vi "Simulated VeriStand Engine.PCL.vi"(8 "error in (no error)":errorcluster, 11 "Simulated VeriStand Engine in":refnum<class "Simulated VeriStand Engine.lvclass">) -> (0 "error out":errorcluster, 3 "Simulated VeriStand Engine out":refnum<class "Simulated VeriStand Engine.lvclass">)   [LabVIEW 2016, in "Simulated VeriStand Engine.lvclass"]
uses:
  Simulated VeriStand Engine.lvclass
  Simulated VeriStand Engine.lvclass/Simulated VeriStand Engine.ctl
  Simulated VeriStand Engine Interface/Simulated VeriStand Engine.Interface.lvclass/Simulated VeriStand Engine.Interface.ctl
  Source/Submodules/Memory/Source/Classes/Pointer/Memory.Pointer.lvclass/Memory.Pointer.ctl
  Accessors/Simulated VeriStand Engine.Get Interface.vi
  Simulated VeriStand Engine Interface/Methods/Simulated VeriStand Engine.Interface.Read.vi
  Simulated VeriStand Engine Interface/Methods/Simulated VeriStand Engine.Interface.Read.Stop.vi
  Source/Submodules/Memory/Source/Classes/Pointer/Memory.Pointer.Read.vi
  Source/Submodules/Memory/Source/Classes/Pointer/Memory.Pointer.Read.Safe.0D.Bool.vi
  Simulated VeriStand Engine Interface/Accessors/Simulated VeriStand Engine.Interface.Get Pointers.vi
  Simulated VeriStand Engine Interface/Accessors/Simulated VeriStand Engine.Interface.Get Control Pointers.vi
  Source/Submodules/Memory/Source/Classes/Pointer/Memory.Pointer.Read.Unsafe.0D.Bool.vi
  Source/Submodules/Memory/Source/Classes/Pointer/Memory.Pointer.Parameter Check.Null Pointer.vi
  Source/Submodules/Memory/Source/Classes/Pointer/Memory.Pointer.Parameter Check.Subset.vi
  Source/Submodules/Memory/Source/Classes/Pointer/Memory.Pointer.Get Address.vi
  Source/Submodules/Memory/Source/Classes/Pointer/Memory.Pointer.Errors.vi
  Source/Submodules/Memory/Source/Classes/Pointer/Memory.Pointer.Errors.Null Pointer.vi
  Source/Submodules/Memory/Source/Classes/Pointer/Memory.Pointer.Errors.Out of Bounds.vi
  Source/Submodules/Memory/Source/Classes/Pointer/Memory.Pointer.Get Size.vi
  Source/Submodules/Memory/Source/Classes/Pointer/Memory.Pointer.Errors.Create Error.vi
  Source/Submodules/Memory/Source/Submodules/SEH/Source/VIs/Static Error Handling.Source Buffer.Write.String.vi
  Source/Submodules/Memory/Source/Classes/Pointer/Memory.Pointer.Errors.Write Pointer Size.vi
  Source/Submodules/Memory/Source/Submodules/SEH/Source/VIs/Static Error Handling.Source Buffer.Write.Numeric.Scalar.Base10.vi
  Source/Submodules/Memory/Source/Submodules/SEH/Source/VIs/Static Error Handling.Source Buffer.Write.Numeric.Scalar.Base10 (U64).vi
  Source/Submodules/Memory/Source/Submodules/SEH/Source/VIs/Static Error Handling.Error Cluster Constant.vi
  Source/Submodules/Memory/Source/Submodules/SEH/Source/VIs/Static Error Handling.Error Cluster Constant (256B).vi
  Source/Submodules/Memory/Source/Submodules/SEH/Source/VIs/Static Error Handling.Parameters.Status.Set.vi
  Source/Submodules/Memory/Source/Submodules/SEH/Source/VIs/Static Error Handling.Parameters.Code.Set.vi
  Source/Submodules/Memory/Source/Submodules/SEH/Source/VIs/Static Error Handling.Parameters.VI Source.Set.vi
  Source/Submodules/Memory/Source/Constants/Memory.Constants.vi
  Source/Submodules/Memory/Source/Constants/Memory.Constants.Library Name.vi
  Source/Submodules/Memory/Source/Classes/Pointer/Memory.Pointer.Errors.Get Info.vi
  Source/Submodules/Memory/Source/Classes/Internal/Memory.Pointer.Internal.lvclass
  C:/Git/Sourcetree/DSF/Source/Submodules/Memory/Source/Classes/Pointer/Memory.Pointer.lvclass
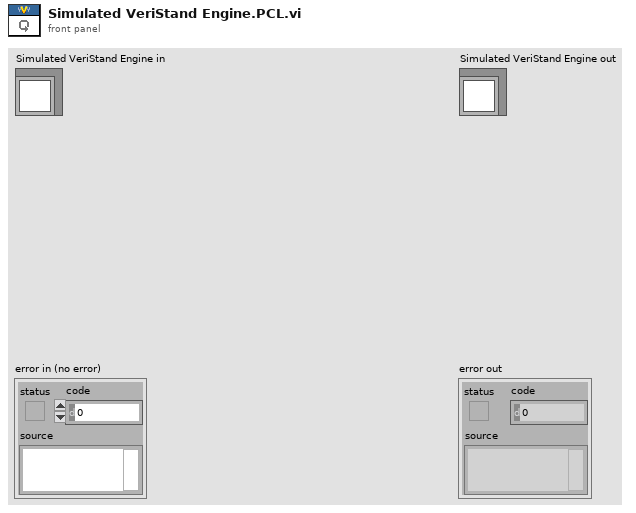
[diagram p1: front panel]
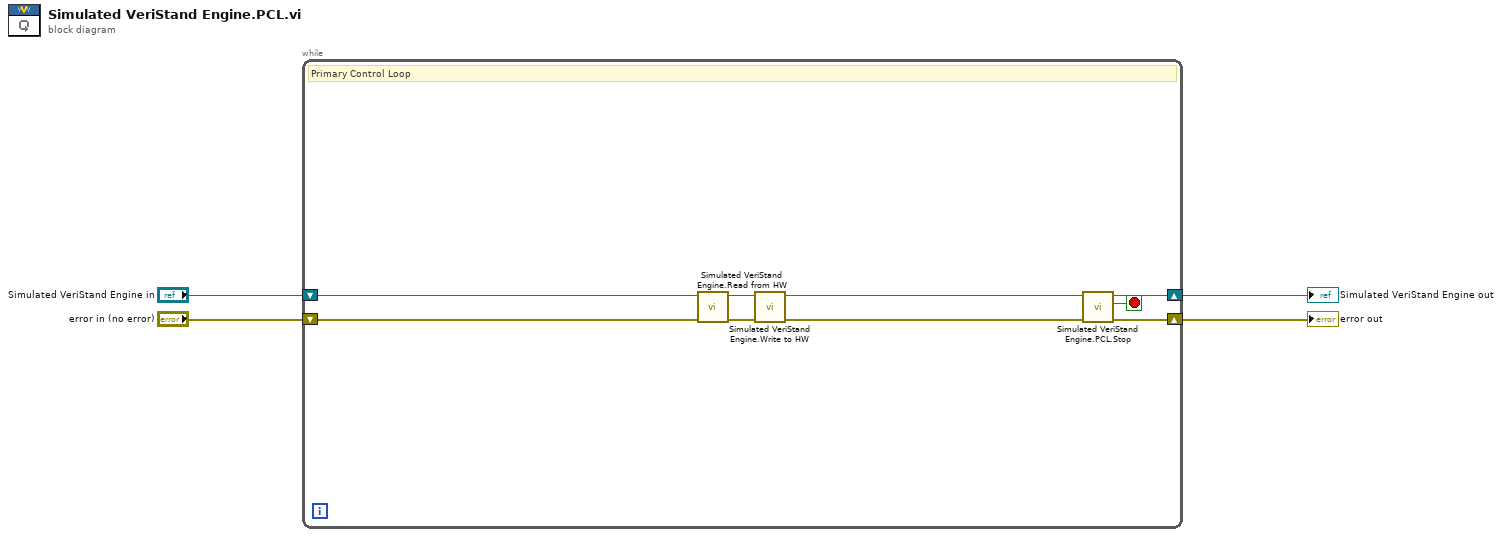
[diagram p0: block diagram]
diagram:
  n1 = while {
    shift-right: [w7] -> w1
    shift-left: "Simulated VeriStand Engine in" -> [w11]
    shift-right: [w6] -> w2
    shift-left: "error in (no error)" -> [w10]
    stop <- w5 stop-if-true
    # "Primary Control Loop"
    n2 = call-dynamic "Simulated VeriStand Engine.Read from HW.vi"("error in (no error)"=w10, "Simulated VeriStand Engine in"=w11) -> ("error out"=w13:errorcluster, "Simulated VeriStand Engine out"=w12:refnum<class "Simulated VeriStand Engine.lvclass">)  [unwired: 8 in]
    n3 = call-dynamic "Simulated VeriStand Engine.Write to HW.vi"("error in (no error)"=w13, "Simulated VeriStand Engine in"=w12) -> ("error out"=w8:errorcluster, "Simulated VeriStand Engine out"=w9:refnum<class "Simulated VeriStand Engine.lvclass">)  [unwired: 8 in]
    n4 = call "Simulated VeriStand Engine.PCL.Stop.vi"("error in (no error)"=w8, "Simulated VeriStand Engine in"=w9) -> ("error out"=w6:errorcluster, "stop"=w5:bool, "Simulated VeriStand Engine out"=w7:refnum<class "Simulated VeriStand Engine.lvclass">)  [unwired: 7 in]
  }
  "error out" <- w2
  "Simulated VeriStand Engine out" <- w1
